vi "BMU诊断标定.vi"(5 "timeout":u32, 6 "Socket":dbl, 7 "通用配置?":bool, 8 "CAN端口":u16(ring), 9 "设备索引号":u16(ring), 10 "CAN卡类型":u32(ring)=21, 11 "从板号":u8=1) -> (3 "成功?":bool)   [LabVIEW 2013] (continued)
            n2234 = stacked-sequence {
              tunnel: w2894 -> [_ w2901 w2905]
              tunnel: w2893 -> [_ w2900 w2904]
              frame #0 {
                n2235 = local write "项目信息"(string[][] [] ("项目信息")) -> ()
              }
              frame #1 {
                n2236 = call "表格数据输入-8.6.vi"("行数"=u32 0, "列数"=u32 0, "字符串数组"=w2900, "表格引用"=w2901) -> ()  [unwired: 8 out]
              }
              frame #2 {
                n2237 = Array Size(array=w2904) -> (size(s)=w2903:i32)
                n2238 = for {
                  N: w2903 -> [_]
                  tunnel: [""] -> w2902 mode=indexing
                }
                n2239 = call "表格数据输入-8.6.vi"("行数"=u32 0, "列数"=u32 1, "字符串数组"=w2902, "表格引用"=w2905) -> ()  [unwired: 8 out]
              }
            }
          }
          event "主界面选项": Value Change {
            n2240 = event-data() -> ("NewVal"=w2909:enum32{"单选选项1", "单选选项2", "单选选项2 2", "单选选项2 3"})  [unwired: 6 out]
            n2241 = control-ref of="单选选项2 2"() -> (w2914:refnum<vi>)
            n2242 = control-ref of="单选选项2"() -> (w2916:refnum<vi>)
            n2243 = control-ref of="单选选项1"() -> (w2915:refnum<vi>)
            n2244 = control-ref of="单选选项2 3"() -> (w2910:refnum<vi>)
            n2245 = Build Array(w2915, w2916, w2914, w2910) -> (w2913:refnum<vi>[])
            n2246 = case shown="\"单选选项2 3\"" w2909 {
              selector: w2909 -> [w2927 w2932 w2937 w2942]
              tunnel: w2913 -> [w2928 w2933 w2938 w2943]
              tunnel: [w2926 w2931 w2936 w2941] -> w2919
              tunnel: [w2925 w2930 w2935 w2940] -> w2918
              tunnel: [enum32{"读写参数", "版本读取", "其它诊断"}."读写参数" ("选项卡控件 2") enum32{"读写参数", "版本读取", "其它诊断"}."版本读取" ("选项卡控件 2") enum32{"读写参数", "版本读取", "其它诊断"}."其它诊断" ("选项卡控件 2") enum32{"读写参数", "版本读取", "其它诊断", "高压板校正"}."高压板校正" ("选项卡控件 2")] -> w2917
              frame "单选选项1", Default {
                n2247 = Delete From Array(array=w2928, index=w2927) -> (deleted portion=w2925:refnum<vi>, array with subset deleted=w2926:refnum<vi>[])  [unwired: 1 in]
              }
              frame "单选选项2" {
                n2248 = Delete From Array(array=w2933, index=w2932) -> (deleted portion=w2930:refnum<vi>, array with subset deleted=w2931:refnum<vi>[])  [unwired: 1 in]
              }
              frame "单选选项2 2" {
                n2249 = Delete From Array(array=w2938, index=w2937) -> (deleted portion=w2935:refnum<vi>, array with subset deleted=w2936:refnum<vi>[])  [unwired: 1 in]
              }
              frame "单选选项2 3" {
                n2250 = Delete From Array(array=w2943, index=w2942) -> (deleted portion=w2940:refnum<vi>, array with subset deleted=w2941:refnum<vi>[])  [unwired: 1 in]
              }
            }
            n2251 = local write "面板选择"(w2917) -> ()
            n2252 = for {
              tunnel: u32 16777215 -> [w2923]
              tunnel: w2919 -> [w2922] mode=indexing
              n2253 = property class="Bool (严格)"(reference=w2922, "BoolText.TextColor"=w2923) -> ()  [unwired: 1 in, 2 out]
            }
            n2254 = property class="Bool (严格)"(reference=w2918, "BoolText.TextColor"=u32 65511) -> ()  [unwired: 1 in, 2 out]
          }
          event "主从板": Value Change {
            w2945 = FALSE ("可见")
            n2255 = event-data() -> ()  [unwired: 7 out]
            n2256 = control-ref of="单选选项2"() -> (w2953:refnum<vi>)
            n2257 = control-ref of="单选选项1"() -> (w2952:refnum<vi>)
            n2258 = local read "主从板"() -> (w2960:enum32{"单选选项2", "单选选项1"})
            n2259 = Build Array(w2953, w2952) -> (w2959:refnum<vi>[])
            n2260 = case shown="\"单选选项2\"" w2960 {
              selector: w2960 -> [w3005 w3048]
              tunnel: w2959 -> [w3006 w3047]
              tunnel: [enum32{"主板", "从板"}."主板" ("主从选择") enum32{"主板", "从板"}."从板" ("主从选择")] -> w2958
              tunnel: [w3004 w3046] -> w2955
              tunnel: [w3003 w3045] -> w2954
              tunnel: [TRUE FALSE] -> w2950
              tunnel: [w2964 w3025] -> w2947
              tunnel: [w2965 w3030] -> w2946
              tunnel: [FALSE ("可见") TRUE ("可见")] -> w2944
              frame "单选选项1", Default {
                n2261 = global read "功能码全局.vi" "主板项目信息7"() -> (w2976:bool[])
                n2262 = global read "功能码全局.vi" "主板项目信息4"() -> (w2999:bool[])
                n2263 = global read "功能码全局.vi" "主板控制类信息10"() -> (w2980:bool[])
                n2264 = global read "功能码全局.vi" "主板故障阀值9"() -> (w2977:bool[])
                n2265 = global read "功能码全局.vi" "主板项目信息5"() -> (w2990:bool[])
                n2266 = global read "功能码全局.vi" "主板项目信息6"() -> (w3000:bool[])
                n2267 = global read "功能码全局.vi" "主板版本号11"() -> (w2991:bool[])
                n2268 = Delete From Array(array=w3000, length=1 ("长度"), index=0 ("索引")) -> (deleted portion=w2989:bool[], array with subset deleted=w2972:bool[])
                n2269 = Index Array(array=w2999, index #1=5 ("索引"), index #2=6 ("索引")) -> (element #1=w2988:bool, element #2=w2971:bool)
                n2270 = Index Array(array=w2991) -> (element #1=w2984:bool, element #2=w2967:bool)  [unwired: 2 in]
                n2271 = Array Subset(array=w2977, index=2 ("索引"), length=3 ("长度")) -> (w2986:bool[])
                n2272 = Delete From Array(array=w2976, length=3 ("索引"), index=2 ("长度")) -> (deleted portion=w2987:bool[], array with subset deleted=w2970:bool[])
                n2273 = Array Subset(array=w2980, index=4 ("索引"), length=2 ("长度")) -> (w2985:bool[])
                n2274 = Delete From Array(array=w3006, index=w3005) -> (deleted portion=w3003:refnum<vi>, array with subset deleted=w3004:refnum<vi>[])  [unwired: 1 in]
                n2275 = Insert Into Array(array=w2990, new element #1=w2989, new element #2=w2988, new element #3=w2987, new element #4=w2986, new element #5=w2985, new element #6=w2984) -> (w2983:bool[])  [unwired: 1 in]
                n2276 = Array Subset(array=w2980, index=6 ("索引"), length=2 ("长度")) -> (w2968:bool[])
                n2277 = Array Subset(array=w2977, index=5 ("索引"), length=3 ("长度")) -> (w2969:bool[])
                n2278 = And Array Elements(Boolean array=w2983) -> (logical AND=w2965:bool)
                n2279 = Insert Into Array(array=w2972, new element #1=w2971, new element #2=w2970, new element #3=w2969, new element #4=w2968, new element #5=w2967) -> (w2966:bool[])  [unwired: 1 in]
                n2280 = And Array Elements(Boolean array=w2966) -> (logical AND=w2964:bool)
              }
              frame "单选选项2" {
                n2281 = global read "功能码全局.vi" "18"() -> (w3021:bool[])
                n2282 = global read "功能码全局.vi" "15"() -> (w3042:bool[])
                n2283 = global read "功能码全局.vi" "16"() -> (w3039:bool[])
                n2284 = Delete From Array(array=w3047, index=w3048) -> (deleted portion=w3045:refnum<vi>, array with subset deleted=w3046:refnum<vi>[])  [unwired: 1 in]
                n2285 = Index Array(array=w3039, index #1=4 ("索引"), index #2=5 ("索引"), index #3=6 ("索引"), index #4=7 ("索引")) -> (element #1=w3033:bool, element #2=w3032:bool, element #3=w3028:bool, element #4=w3027:bool)
                n2286 = Index Array(array=w3021, index #1=4 ("索引"), index #2=5 ("索引"), index #3=6 ("索引"), index #4=7 ("索引"), index #5=2 ("索引"), index #6=3 ("索引"), index #7=0 ("索引"), index #8=1 ("索引")) -> (element #1=w3014:bool, element #2=w3017:bool, element #3=w3016:bool, element #4=w3015:bool, element #5=w3013:bool, element #6=w3012:bool, element #7=w3007:bool, element #8=w3008:bool)
                n2287 = Delete From Array(array=w3042, length=4 ("长度"), index=0 ("索引")) -> (deleted portion=w3034:bool[], array with subset deleted=w3029:bool[])
                n2288 = Insert Into Array(array=w3029, new element #1=w3028, new element #2=w3027, new element #3=w3017, new element #4=w3016, new element #5=w3015, new element #6=w3008) -> (w3026:bool[])  [unwired: 1 in]
                n2289 = Insert Into Array(array=w3034, new element #1=w3033, new element #2=w3032, new element #3=w3014, new element #4=w3013, new element #5=w3012, new element #6=w3007) -> (w3031:bool[])  [unwired: 1 in]
                n2290 = And Array Elements(Boolean array=w3031) -> (logical AND=w3030:bool)
                n2291 = And Array Elements(Boolean array=w3026) -> (logical AND=w3025:bool)
              }
            }
            n2292 = property on="全部写入" class="Bool (严格)"("Visible"=w2947) -> ()  [unwired: 2 in, 2 out]
            n2293 = property on="全部读取" class="Bool (严格)"("Visible"=w2946) -> ()  [unwired: 2 in, 2 out]
            n2294 = property on="从板号" class="DigNum (严格)"("Visible"=w2944) -> ()  [unwired: 2 in, 2 out]
            n2295 = local write "主从选择"(w2958) -> ()
            n2296 = property on="从板个数" class="DigNum (严格)"("Visible"=w2950) -> ()  [unwired: 2 in, 2 out]
            n2297 = for {
              tunnel: u32 87470 -> [w2962]
              tunnel: w2955 -> [w2961] mode=indexing
              n2298 = property class="Bool (严格)"(reference=w2961, "BoolText.TextColor"=w2962) -> ()  [unwired: 1 in, 2 out]
            }
            n2299 = Not(x=w2950) -> (.not. x?=w2951:bool)
            n2300 = property class="Bool (严格)"(reference=w2954, "BoolText.TextColor"=u32 16777215) -> ()  [unwired: 1 in, 2 out]
            n2301 = property on="主板选项" class="Tree (严格)"("Visible"=w2950) -> ()  [unwired: 2 in, 2 out]
            n2302 = property on="从板选项" class="Tree (严格)"("Visible"=w2951) -> ()  [unwired: 2 in, 2 out]
            n2303 = property on="当前从板板号" class="DigNum (严格)"("Visible"=w2951) -> ()  [unwired: 2 in, 2 out]
            n2304 = property on="单个读取" class="Bool (严格)"("Visible"=w2945) -> ()  [unwired: 2 in, 2 out]
            n2305 = property on="单个写入" class="Bool (严格)"("Visible"=w2945) -> ()  [unwired: 2 in, 2 out]
          }
          event "从板号": Value Change {
            n2306 = event-data() -> ()  [unwired: 7 out]
            n2307 = local read "key names"() -> (w3050:string[])
            n2308 = Empty Array?(array=w3050) -> (empty?=w3049:bool)
            n2309 = case shown="假" w3049 {
              tunnel: w3050 -> [w3053 _]
              frame False {
                n2310 = stacked-sequence {
                  seq-local: [w3054 _] -> [_ w3117]
                  tunnel: w3053 -> [w3062 _]
                  frame #0 {
                    w3093 = 2 ("长度")
                    w3090 = 20 ("长度")
                    w3078 = 1 ("索引")
                    n2311 = local read "从板号"() -> (w3054:u8)
                    n2312 = local read "输出数组"() -> (w3063:string[][])
                    n2313 = Decrement(x=w3054) -> (x-1=w3060:u8)
                    n2314 = Index Array(array=w3063, index (col)=w3060) -> (element=w3091:string[])  [unwired: 1 in]
                    n2315 = global write "读配置文件全局2.vi" "从板板号"(w3054) -> ()
                    n2316 = Search 1D Array(1D array=w3062, element="风机开启温度" ("元素")) -> (index of element=w3075:i32)  [unwired: 1 in]
                    n2317 = Search 1D Array(1D array=w3062, element="电压过高一级" ("元素"), start index (0)=w3075) -> (index of element=w3073:i32)
                    n2318 = Decrement(x=w3075) -> (x-1=w3077:i32)
                    n2319 = Array Subset(array=w3091, index=w3078, length=w3077) -> (w3061:string[])
                    n2320 = Array Subset(array=w3091, index=w3073, length=21 ("长度")) -> (w3065:string[])
                    n2321 = Array Subset(array=w3062, index=w3078, length=w3077) -> (w3108:string[])
                    n2322 = Array Subset(array=w3091, index=w3075, length=7 ("长度")) -> (w3071:string[])
                    n2323 = for {
                      tunnel: w3065 -> [w3110] mode=indexing
                      tunnel: [w3109] -> w3064 mode=indexing
                      n2324 = Fract/Exp String To Number(string=w3110) -> (number=w3109:dbl)  [unwired: 3 in, 1 out]
                    }
                    n2325 = for {
                      tunnel: w3071 -> [w3112] mode=indexing
                      tunnel: [w3111] -> w3055 mode=indexing
                      n2326 = Fract/Exp String To Number(string=w3112) -> (number=w3111:dbl)  [unwired: 3 in, 1 out]
                    }
                    n2327 = Delete From Array(array=w3064, length=7 ("长度"), index=0 ("索引")) -> (deleted portion=w3058:dbl[], array with subset deleted=w3068:dbl[])
                    n2328 = Array To Cluster(array=w3055) -> (cluster=w3080:T20)
                    n2329 = global write "读配置文件全局2.vi" "加热控制参数"(w3055) -> ()
                    n2330 = Delete From Array(array=w3068, length=7 ("长度"), index=0 ("索引")) -> (deleted portion=w3057:dbl[], array with subset deleted=w3056:dbl[])
                    n2331 = local write "加热控制参数"(w3080) -> ()
                    n2332 = Array To Cluster(array=w3058) -> (cluster=w3105:T20)
                    n2333 = Array To Cluster(array=w3056) -> (cluster=w3107:T20)
                    n2334 = Array To Cluster(array=w3057) -> (cluster=w3106:T20)
                    n2335 = global write "读配置文件全局2.vi" "三级故障阀值"(w3056) -> ()
                    n2336 = global write "读配置文件全局2.vi" "一级故障阀值"(w3058) -> ()
                    n2337 = global write "读配置文件全局2.vi" "二级故障阀值"(w3057) -> ()
                    n2338 = local write "一级故障 6"(w3105) -> ()
                    n2339 = local write "一级故障 8"(w3107) -> ()
                    n2340 = local write "一级故障 7"(w3106) -> ()
                    n2341 = Search 1D Array(1D array=w3108, element="温度个数" ("元素")) -> (index of element=w3087:i32)  [unwired: 1 in]
                    n2342 = Search 1D Array(1D array=w3108, element="第一个保险通道" ("元素")) -> (index of element=w3088:i32)  [unwired: 1 in]
                    n2343 = Search 1D Array(1D array=w3108, element="电压个数" ("元素")) -> (index of element=w3086:i32)  [unwired: 1 in]
                    n2344 = Search 1D Array(1D array=w3108, element="第1通道电压个数" ("元素")) -> (index of element=w3089:i32)  [unwired: 1 in]
                    n2345 = Array Subset(array=w3061, index=w3086, length=2 ("长度")) -> (w3094:string[])
                    n2346 = Array Subset(array=w3061, index=w3087, length=w3093) -> (w3096:string[])
                    n2347 = Array Subset(array=w3061, index=w3088, length=20 ("长度")) -> (w3097:string[])
                    n2348 = Array Subset(array=w3061, index=w3089, length=w3090) -> (w3095:string[])
                    n2349 = Insert Into Array(array=w3094, new element #1=w3095, new element #2=w3096, new element #3=w3097) -> (w3059:string[])  [unwired: 1 in]
                    n2350 = Array Subset(array=w3108, index=w3086, length=w3093) -> (w3098:string[])
                    n2351 = Array Subset(array=w3108, index=w3087, length=w3093) -> (w3100:string[])
                    n2352 = Array Subset(array=w3108, index=w3088, length=w3090) -> (w3101:string[])
                    n2353 = Array Subset(array=w3108, index=w3089, length=w3090) -> (w3099:string[])
                    n2354 = global write "读配置文件全局2.vi" "表格"(w3059) -> ()
                    n2355 = Insert Into Array(array=w3098, new element #1=w3099, new element #2=w3100, new element #3=w3101) -> (w3103:string[])  [unwired: 1 in]
                    n2356 = Build Array(w3103, w3059) -> (w3102:string[][])
                    n2357 = Transpose 2D Array(2D array=w3102) -> (transposed array=w3104:string[][])
                    n2358 = local write "项目信息 2"(w3104) -> ()
                  }
                  frame #1 {
                    n2359 = Number To Decimal String(number=w3117) -> (decimal integer string=w3115:string)  [unwired: 1 in]
                    n2360 = control-ref of="结果"() -> (w3120:refnum<vi>)
                    n2361 = Concatenate Strings("从板", w3115, "导入完成") -> (w3113:string)
                    n2362 = Build Array(w3113) -> (w3118:string[])
                    n2363 = call "表格编辑.vi"("新元素/子数组"=w3118, "活动单元格:单元格背景色"=u32 6618880, "MCListbox引用句柄"=w3120) -> ()  [unwired: 9 out]
                  }
                }
              }
              frame True {
              }
            }
          }
          event "读配置文件": Value Change {
            n2364 = event-data() -> ("NewVal"=w3121:bool)  [unwired: 6 out]
            n2365 = case shown="真" w3121 {
              tunnel: w3125 -> [w3127 w3133]
              tunnel: [w3127 w3132] -> w3124
              tunnel: w3123 -> [w3126 w3131]
              tunnel: [w3126 w3130] -> w3122
              frame False {
              }
              frame True {
                n2366 = local write "布尔"(TRUE ("布尔")) -> ()
                n2367 = Enqueue Element(queue=w3133, element="读配置文件", error in (no error)=w3131) -> (queue out=w3132:refnum<queue>, error out=w3130:errorcluster)  [unwired: 2 out]
              }
            }
          }
          event "保存主板参数": Value Change {
            n2368 = event-data() -> ("NewVal"=w3134:bool)  [unwired: 6 out]
            n2369 = case shown="真" w3134 {
              tunnel: w3138 -> [w3140 w3145]
              tunnel: [w3140 w3144] -> w3137
              tunnel: w3136 -> [w3139 w3143]
              tunnel: [w3139 w3142] -> w3135
              frame False {
              }
              frame True {
                n2370 = call <vilib>:"Set Busy.vi"() -> ()  [unwired: 4 in, 8 out]
                n2371 = Enqueue Element(queue=w3145, element="写配置文件", error in (no error)=w3143) -> (queue out=w3144:refnum<queue>, error out=w3142:errorcluster)  [unwired: 2 out]
              }
            }
          }
          event "继电器全开": Value Change {
            n2372 = event-data() -> ("NewVal"=w3146:bool)  [unwired: 6 out]
            n2373 = case shown="真" w3146 {
              tunnel: w3146 -> [_ w3149]
              frame False {
              }
              frame True {
                n2374 = stacked-sequence {
                  tunnel: w3149 -> [_ w3159 _]
                  frame #0 {
                    w3150 = FALSE ("清BUFF")
                    n2375 = local write "正级继电器"(w3150) -> ()
                    n2376 = local write "负级继电器"(w3150) -> ()
                    n2377 = local write "充电继电器"(w3150) -> ()
                    n2378 = local write "加热继电器"(w3150) -> ()
                    n2379 = local write "风机继电器"(w3150) -> ()
                    n2380 = local write "预充电继电器"(w3150) -> ()
                    n2381 = local write "继电器超时处理"(FALSE ("继电器超时处理")) -> ()
                    n2382 = local write "主从选择"(enum32{"主板", "从板"}."主板" ("主从选择")) -> ()
                    n2383 = local write "清BUFF"(FALSE ("清BUFF")) -> ()
                  }
                  frame #1 {
                    n2384 = case shown="真" w3159 {
                      selector: w3159 -> [_ w3174]
                      frame False {
                      }
                      frame True {
                        w3170 = 256.0 ("y")
                        w3161 = u32 1 ("命令序号")
                        w3160 = u8 192 ("命令")
                        n2385 = local read "动作保持时间"() -> (w3171:dbl)
                        n2386 = Quotient & Remainder(x=w3171, y=w3170) -> (x-y*floor(x/y)=w3163:dbl, floor(x/y)=w3167:dbl)
                        n2387 = Quotient & Remainder(x=w3167, y=w3170) -> (x-y*floor(x/y)=w3164:dbl, floor(x/y)=w3168:dbl)
                        n2388 = Quotient & Remainder(x=w3168, y=w3170) -> (x-y*floor(x/y)=w3165:dbl, floor(x/y)=w3169:dbl)
                        n2389 = local read "设备索引号"() -> (w3178:u16)
                        n2390 = local read "CAN卡类型"() -> (w3179:u32)
                        n2391 = local read "CAN端口"() -> (w3177:u16)
                        n2392 = Boolean To (0,1)(Boolean=w3174) -> (0, 1=w3172:i16)
                        n2393 = Quotient & Remainder(x=w3169, y=w3170) -> (x-y*floor(x/y)=w3166:dbl)  [unwired: 1 out]
                        n2394 = Build Array(i16 170 ("元素"), w3172, w3166, w3165, w3164, w3163, 0.0 ("元素")) -> (w3175:dbl[])
                        n2395 = call "多帧发送机制(EV05).vi"("can卡类型"=w3179, "设备索引号"=w3178, "CAN端口"=w3177, "命令"=w3160, "板号"=u8 0, "命令序号"=w3161, "输入数据"=w3175) -> ()  [unwired: 2 in, 11 out]
                        n2396 = local write "命令序号"(w3161) -> ()
                        n2397 = local write "命令"(w3160) -> ()
                      }
                    }
                    n2398 = local write "控制1"(TRUE ("控制1")) -> ()
                    n2399 = local write "写?"(FALSE ("写?")) -> ()
                    n2400 = local write "消除"(TRUE ("消除")) -> ()
                    n2401 = global write "EV05全局变量1.vi" "流控帧 2"(TRUE ("流控帧 2")) -> ()
                    n2402 = global write "EV05全局变量1.vi" "流控帧"(FALSE ("流控帧")) -> ()
                  }
                  frame #2 {
                    n2403 = flat-sequence {
                      tunnel: [w3181] -> w3180
                      tunnel: w3180 -> [w3188]
                      frame #0 {
                        n2404 = while {
                          tunnel: [w3182] -> w3181
                          i -> [w3186]
                          stop <- w3183 stop-if-true
                          n2405 = local read "继电器超时处理"() -> (w3182:bool)
                          n2406 = Greater Or Equal?(x=w3186, y=20) -> (x >= y?=w3184:bool)
                          n2407 = Wait Until Next ms Multiple(millisecond multiple=u32 100 ("毫秒倍数")) -> ()  [unwired: 1 out]
                          n2408 = Or(x=w3182, y=w3184) -> (x .or. y?=w3183:bool)
                        }
                      }
                      frame #1 {
                        n2409 = case shown="真" w3188 {
                          frame False {
                            n2410 = One Button Dialog(message="继电器处理超时" ("消息"), button name ("OK")="是" ("按钮名称（“确定”）")) -> ()  [unwired: 1 out]
                          }
                          frame True {
                            w3191 = TRUE ("清BUFF")
                            n2411 = local write "正级继电器"(w3191) -> ()
                            n2412 = local write "负级继电器"(w3191) -> ()
                            n2413 = local write "充电继电器"(w3191) -> ()
                            n2414 = local write "加热继电器"(w3191) -> ()
                            n2415 = local write "风机继电器"(w3191) -> ()
                            n2416 = local write "预充电继电器"(w3191) -> ()
                          }
                        }
                      }
                    }
                  }
                }
              }
            }
          }
          event "继电器全关": Value Change {
            n2417 = event-data() -> ("NewVal"=w3192:bool)  [unwired: 6 out]
            n2418 = case shown="真" w3192 {
              tunnel: w3192 -> [_ w3195]
              frame False {
              }
              frame True {
                n2419 = stacked-sequence {
                  tunnel: w3195 -> [_ w3205 _]
                  frame #0 {
                    w3196 = TRUE ("清BUFF")
                    n2420 = local write "正级继电器"(w3196) -> ()
                    n2421 = local write "负级继电器"(w3196) -> ()
                    n2422 = local write "充电继电器"(w3196) -> ()
                    n2423 = local write "加热继电器"(w3196) -> ()
                    n2424 = local write "风机继电器"(w3196) -> ()
                    n2425 = local write "预充电继电器"(w3196) -> ()
                    n2426 = local write "继电器超时处理"(FALSE ("继电器超时处理")) -> ()
                    n2427 = local write "主从选择"(enum32{"主板", "从板"}."主板" ("主从选择")) -> ()
                    n2428 = global write "EV05全局变量1.vi" "流控帧"(FALSE ("流控帧")) -> ()
                    n2429 = local write "清BUFF"(FALSE ("清BUFF")) -> ()
                  }
                  frame #1 {
                    n2430 = case shown="真" w3205 {
                      selector: w3205 -> [_ w3220]
                      frame False {
                      }
                      frame True {
                        w3216 = 256.0 ("y")
                        w3207 = u32 1 ("命令序号")
                        w3206 = u8 192 ("命令")
                        n2431 = local read "动作保持时间"() -> (w3217:dbl)
                        n2432 = Quotient & Remainder(x=w3217, y=w3216) -> (x-y*floor(x/y)=w3209:dbl, floor(x/y)=w3213:dbl)
                        n2433 = Quotient & Remainder(x=w3213, y=w3216) -> (x-y*floor(x/y)=w3210:dbl, floor(x/y)=w3214:dbl)
                        n2434 = Quotient & Remainder(x=w3214, y=w3216) -> (x-y*floor(x/y)=w3211:dbl, floor(x/y)=w3215:dbl)
                        n2435 = local read "设备索引号"() -> (w3224:u16)
                        n2436 = local read "CAN卡类型"() -> (w3225:u32)
                        n2437 = local read "CAN端口"() -> (w3223:u16)
                        n2438 = Boolean To (0,1)(Boolean=w3220) -> (0, 1=w3218:i16)
                        n2439 = Quotient & Remainder(x=w3215, y=w3216) -> (x-y*floor(x/y)=w3212:dbl)  [unwired: 1 out]
                        n2440 = Build Array(i16 85 ("元素"), w3218, w3212, w3211, w3210, w3209, 0.0 ("元素")) -> (w3221:dbl[])
                        n2441 = call "多帧发送机制(EV05).vi"("can卡类型"=w3225, "设备索引号"=w3224, "CAN端口"=w3223, "命令"=w3206, "板号"=u8 0, "命令序号"=w3207, "输入数据"=w3221) -> ()  [unwired: 2 in, 11 out]
                        n2442 = local write "命令序号"(w3207) -> ()
                        n2443 = local write "命令"(w3206) -> ()
                      }
                    }
                    n2444 = local write "控制1"(TRUE ("控制1")) -> ()
                    n2445 = local write "写?"(FALSE ("写?")) -> ()
                    n2446 = local write "消除"(TRUE ("消除")) -> ()
                    n2447 = global write "EV05全局变量1.vi" "流控帧 2"(TRUE ("流控帧 2")) -> ()
                  }
                  frame #2 {
                    n2448 = flat-sequence {
                      tunnel: [w3227] -> w3226
                      tunnel: w3226 -> [w3234]
                      frame #0 {
                        n2449 = while {
                          tunnel: [w3228] -> w3227
                          i -> [w3232]
                          stop <- w3229 stop-if-true
                          n2450 = local read "继电器超时处理"() -> (w3228:bool)
                          n2451 = Greater Or Equal?(x=w3232, y=20) -> (x >= y?=w3230:bool)
                          n2452 = Wait Until Next ms Multiple(millisecond multiple=u32 100 ("毫秒倍数")) -> ()  [unwired: 1 out]
                          n2453 = Or(x=w3228, y=w3230) -> (x .or. y?=w3229:bool)
                        }
                      }
                      frame #1 {
                        n2454 = case shown="真" w3234 {
                          frame False {
                            n2455 = One Button Dialog(message="继电器处理超时" ("消息"), button name ("OK")="是" ("按钮名称（“确定”）")) -> ()  [unwired: 1 out]
                          }
                          frame True {
                            w3237 = FALSE ("清BUFF")
                            n2456 = local write "正级继电器"(w3237) -> ()
                            n2457 = local write "负级继电器"(w3237) -> ()
                            n2458 = local write "充电继电器"(w3237) -> ()
                            n2459 = local write "加热继电器"(w3237) -> ()
                            n2460 = local write "风机继电器"(w3237) -> ()
                            n2461 = local write "预充电继电器"(w3237) -> ()
                          }
                        }
                      }
                    }
                  }
                }
              }
            }
          }
          event "控制按键全为开": Value Change {
            n2462 = event-data() -> ("NewVal"=w3238:bool)  [unwired: 6 out]
            n2463 = case shown="真" w3238 {
              frame False {
              }
              frame True {
                w3239 = TRUE ("正级继电器")
                n2464 = local write "加热继电器(从)"(w3239) -> ()
                n2465 = local write "风机继电器(从)"(w3239) -> ()
                n2466 = local write "DO1 2"(w3239) -> ()
                n2467 = local write "DO1"(w3239) -> ()
                n2468 = local write "DO2"(w3239) -> ()
                n2469 = local write "正级继电器"(w3239) -> ()
                n2470 = local write "负级继电器"(w3239) -> ()
                n2471 = local write "加热继电器"(w3239) -> ()
                n2472 = local write "预充电继电器"(w3239) -> ()
                n2473 = local write "充电继电器"(w3239) -> ()
                n2474 = local write "风机继电器"(w3239) -> ()
              }
            }
          }
          event "控制按键全为关": Value Change {
            n2475 = event-data() -> ("NewVal"=w3240:bool)  [unwired: 6 out]
            n2476 = case shown="真" w3240 {
              frame False {
              }
              frame True {
                w3241 = FALSE ("正级继电器")
                n2477 = local write "加热继电器(从)"(w3241) -> ()
                n2478 = local write "风机继电器(从)"(w3241) -> ()
                n2479 = local write "DO1 2"(w3241) -> ()
                n2480 = local write "DO1"(w3241) -> ()
                n2481 = local write "DO2"(w3241) -> ()
                n2482 = local write "正级继电器"(w3241) -> ()
                n2483 = local write "负级继电器"(w3241) -> ()
                n2484 = local write "加热继电器"(w3241) -> ()
                n2485 = local write "预充电继电器"(w3241) -> ()
                n2486 = local write "充电继电器"(w3241) -> ()
                n2487 = local write "风机继电器"(w3241) -> ()
              }
            }
          }
          event "正级继电器": Value Change {
            n2488 = event-data() -> ("NewVal"=w3242:bool)  [unwired: 6 out]
            n2489 = stacked-sequence {
              tunnel: w3242 -> [_ w3255 _]
              frame #0 {
                w3245 = FALSE ("清BUFF")
                n2490 = local write "继电器超时处理"(FALSE ("继电器超时处理")) -> ()
                n2491 = local write "主从选择"(enum32{"主板", "从板"}."主板" ("主从选择")) -> ()
                n2492 = local write "正级继电器 12"(w3245) -> ()
                n2493 = local write "清BUFF"(w3245) -> ()
              }
              frame #1 {
                n2494 = case shown="假" w3255 {
                  selector: w3255 -> [w3270 w3290]
                  tunnel: [w3269 w3289] -> w3254
                  tunnel: [w3257 w3277] -> w3249
                  frame False {
                    w3265 = 256.0 ("y")
                    w3257 = u32 1 ("命令序号")
                    w3269 = u8 192 ("命令")
                    n2495 = local read "动作保持时间"() -> (w3266:dbl)
                    n2496 = Quotient & Remainder(x=w3266, y=w3265) -> (x-y*floor(x/y)=w3258:dbl, floor(x/y)=w3262:dbl)
                    n2497 = Quotient & Remainder(x=w3262, y=w3265) -> (x-y*floor(x/y)=w3259:dbl, floor(x/y)=w3263:dbl)
                    n2498 = Quotient & Remainder(x=w3263, y=w3265) -> (x-y*floor(x/y)=w3260:dbl, floor(x/y)=w3264:dbl)
                    n2499 = local read "设备索引号"() -> (w3274:u16)
                    n2500 = local read "CAN卡类型"() -> (w3275:u32)
                    n2501 = local read "CAN端口"() -> (w3273:u16)
                    n2502 = Boolean To (0,1)(Boolean=w3270) -> (0, 1=w3267:i16)
                    n2503 = Quotient & Remainder(x=w3264, y=w3265) -> (x-y*floor(x/y)=w3261:dbl)  [unwired: 1 out]
                    n2504 = Build Array(i16 1 ("元素"), w3267, w3261, w3260, w3259, w3258, 0.0 ("元素")) -> (w3271:dbl[])
                    n2505 = call "多帧发送机制(EV05).vi"("can卡类型"=w3275, "设备索引号"=w3274, "CAN端口"=w3273, "命令"=w3269, "板号"=u8 0, "命令序号"=w3257, "输入数据"=w3271) -> ()  [unwired: 2 in, 11 out]
                  }
                  frame True {
                    w3285 = 256.0 ("y")
                    w3277 = u32 1 ("命令序号")
                    w3289 = u8 192 ("命令")
                    n2506 = local read "动作保持时间"() -> (w3286:dbl)
                    n2507 = Quotient & Remainder(x=w3286, y=w3285) -> (x-y*floor(x/y)=w3278:dbl, floor(x/y)=w3282:dbl)
                    n2508 = Quotient & Remainder(x=w3282, y=w3285) -> (x-y*floor(x/y)=w3279:dbl, floor(x/y)=w3283:dbl)
                    n2509 = Quotient & Remainder(x=w3283, y=w3285) -> (x-y*floor(x/y)=w3280:dbl, floor(x/y)=w3284:dbl)
                    n2510 = local read "设备索引号"() -> (w3294:u16)
                    n2511 = local read "CAN卡类型"() -> (w3295:u32)
                    n2512 = local read "CAN端口"() -> (w3293:u16)
                    n2513 = Boolean To (0,1)(Boolean=w3290) -> (0, 1=w3287:i16)
                    n2514 = Quotient & Remainder(x=w3284, y=w3285) -> (x-y*floor(x/y)=w3281:dbl)  [unwired: 1 out]
                    n2515 = Build Array(i16 1 ("元素"), w3287, w3281, w3280, w3279, w3278, 0.0 ("元素")) -> (w3291:dbl[])
                    n2516 = call "多帧发送机制(EV05).vi"("can卡类型"=w3295, "设备索引号"=w3294, "CAN端口"=w3293, "命令"=w3289, "板号"=u8 0, "命令序号"=w3277, "输入数据"=w3291) -> ()  [unwired: 2 in, 11 out]
                  }
                }
                n2517 = local write "命令序号"(w3249) -> ()
                n2518 = local write "命令"(w3254) -> ()
                n2519 = local write "控制1"(TRUE ("控制1")) -> ()
                n2520 = local write "写?"(FALSE ("写?")) -> ()
                n2521 = global write "EV05全局变量1.vi" "流控帧"(FALSE ("流控帧")) -> ()
                n2522 = local write "消除"(TRUE ("消除")) -> ()
                n2523 = global write "EV05全局变量1.vi" "流控帧 2"(TRUE ("流控帧 2")) -> ()
              }
              frame #2 {
                n2524 = flat-sequence {
                  tunnel: [w3297] -> w3296
                  tunnel: w3296 -> [w3304]
                  frame #0 {
                    n2525 = while {
                      tunnel: [w3298] -> w3297
                      i -> [w3302]
                      stop <- w3299 stop-if-true
                      n2526 = local read "继电器超时处理"() -> (w3298:bool)
                      n2527 = Greater Or Equal?(x=w3302, y=20) -> (x >= y?=w3300:bool)
                      n2528 = Wait Until Next ms Multiple(millisecond multiple=u32 100 ("毫秒倍数")) -> ()  [unwired: 1 out]
                      n2529 = Or(x=w3298, y=w3300) -> (x .or. y?=w3299:bool)
                    }
                  }
                  frame #1 {
                    n2530 = case shown="假" w3304 {
                      frame False {
                        n2531 = local read "正级继电器"() -> (w3306:bool)
                        n2532 = Not(x=w3306) -> (.not. x?=w3305:bool)
                        n2533 = local write "正级继电器"(w3305) -> ()
                        n2534 = One Button Dialog(message="继电器处理超时" ("消息"), button name ("OK")="是" ("按钮名称（“确定”）")) -> ()  [unwired: 1 out]
                      }
                      frame True {
                      }
                    }
                  }
                }
              }
            }
          }
          event "负级继电器": Value Change {
            n2535 = event-data() -> ("NewVal"=w3309:bool)  [unwired: 6 out]
            n2536 = stacked-sequence {
              tunnel: w3309 -> [_ w3322 _]
              frame #0 {
                w3312 = FALSE ("继电器超时处理")
                n2537 = local write "继电器超时处理"(w3312) -> ()
                n2538 = local write "正级继电器 2"(w3312) -> ()
                n2539 = local write "主从选择"(enum32{"主板", "从板"}."主板" ("主从选择")) -> ()
              }
              frame #1 {
                n2540 = case shown="假" w3322 {
                  selector: w3322 -> [w3336 w3356]
                  tunnel: [w3335 w3355] -> w3321
                  tunnel: [w3324 w3344] -> w3316
                  frame False {
                    w3332 = 256.0 ("y")
                    w3324 = u32 1 ("命令序号")
                    w3335 = u8 192 ("命令")
                    n2541 = local read "动作保持时间"() -> (w3333:dbl)
                    n2542 = Quotient & Remainder(x=w3333, y=w3332) -> (x-y*floor(x/y)=w3325:dbl, floor(x/y)=w3329:dbl)
                    n2543 = Quotient & Remainder(x=w3329, y=w3332) -> (x-y*floor(x/y)=w3326:dbl, floor(x/y)=w3330:dbl)
                    n2544 = Quotient & Remainder(x=w3330, y=w3332) -> (x-y*floor(x/y)=w3327:dbl, floor(x/y)=w3331:dbl)
                    n2545 = Quotient & Remainder(x=w3331, y=w3332) -> (x-y*floor(x/y)=w3328:dbl)  [unwired: 1 out]
                    n2546 = Boolean To (0,1)(Boolean=w3336) -> (0, 1=w3334:i16)
                    n2547 = local read "设备索引号"() -> (w3341:u16)
                    n2548 = local read "CAN卡类型"() -> (w3342:u32)
                    n2549 = local read "CAN端口"() -> (w3340:u16)
                    n2550 = Build Array(i16 2 ("元素"), w3334, w3328, w3327, w3326, w3325, 0.0 ("元素")) -> (w3338:dbl[])
                    n2551 = call "多帧发送机制(EV05).vi"("can卡类型"=w3342, "设备索引号"=w3341, "CAN端口"=w3340, "命令"=w3335, "板号"=u8 0, "命令序号"=w3324, "输入数据"=w3338) -> ()  [unwired: 2 in, 11 out]
                  }
                  frame True {
                    w3352 = 256.0 ("y")
                    w3344 = u32 1 ("命令序号")
                    w3355 = u8 192 ("命令")
                    n2552 = local read "动作保持时间"() -> (w3353:dbl)
                    n2553 = Quotient & Remainder(x=w3353, y=w3352) -> (x-y*floor(x/y)=w3345:dbl, floor(x/y)=w3349:dbl)
                    n2554 = Quotient & Remainder(x=w3349, y=w3352) -> (x-y*floor(x/y)=w3346:dbl, floor(x/y)=w3350:dbl)
                    n2555 = Quotient & Remainder(x=w3350, y=w3352) -> (x-y*floor(x/y)=w3347:dbl, floor(x/y)=w3351:dbl)
                    n2556 = Quotient & Remainder(x=w3351, y=w3352) -> (x-y*floor(x/y)=w3348:dbl)  [unwired: 1 out]
                    n2557 = Boolean To (0,1)(Boolean=w3356) -> (0, 1=w3354:i16)
                    n2558 = local read "设备索引号"() -> (w3361:u16)
                    n2559 = local read "CAN卡类型"() -> (w3362:u32)
                    n2560 = local read "CAN端口"() -> (w3360:u16)
                    n2561 = Build Array(i16 2 ("元素"), w3354, w3348, w3347, w3346, w3345, 0.0 ("元素")) -> (w3358:dbl[])
                    n2562 = call "多帧发送机制(EV05).vi"("can卡类型"=w3362, "设备索引号"=w3361, "CAN端口"=w3360, "命令"=w3355, "板号"=u8 0, "命令序号"=w3344, "输入数据"=w3358) -> ()  [unwired: 2 in, 11 out]
                  }
                }
                n2563 = local write "命令"(w3321) -> ()
                n2564 = local write "命令序号"(w3316) -> ()
                n2565 = local write "清BUFF"(FALSE ("清BUFF")) -> ()
                n2566 = global write "EV05全局变量1.vi" "流控帧"(FALSE ("流控帧")) -> ()
                n2567 = local write "控制1"(TRUE ("控制1")) -> ()
                n2568 = global write "EV05全局变量1.vi" "流控帧 2"(TRUE ("流控帧 2")) -> ()
                n2569 = local write "写?"(FALSE ("写?")) -> ()
                n2570 = local write "消除"(TRUE ("消除")) -> ()
              }
              frame #2 {
                n2571 = flat-sequence {
                  tunnel: [w3364] -> w3363
                  tunnel: w3363 -> [w3371]
                  frame #0 {
                    n2572 = while {
                      tunnel: [w3365] -> w3364
                      i -> [w3369]
                      stop <- w3366 stop-if-true
                      n2573 = local read "继电器超时处理"() -> (w3365:bool)
                      n2574 = Greater Or Equal?(x=w3369, y=20) -> (x >= y?=w3367:bool)
                      n2575 = Wait Until Next ms Multiple(millisecond multiple=u32 100 ("毫秒倍数")) -> ()  [unwired: 1 out]
                      n2576 = Or(x=w3365, y=w3367) -> (x .or. y?=w3366:bool)
                    }
                  }
                  frame #1 {
                    n2577 = case shown="假" w3371 {
                      frame False {
                        n2578 = local read "负级继电器"() -> (w3372:bool)
                        n2579 = Not(x=w3372) -> (.not. x?=w3373:bool)
                        n2580 = local write "负级继电器"(w3373) -> ()
                        n2581 = One Button Dialog(message="继电器处理超时" ("消息"), button name ("OK")="是" ("按钮名称（“确定”）")) -> ()  [unwired: 1 out]
                      }
                      frame True {
                      }
                    }
                  }
                }
              }
            }
          }
          event "预充电继电器": Value Change {
            n2582 = event-data() -> ("NewVal"=w3376:bool)  [unwired: 6 out]
            n2583 = stacked-sequence {
              tunnel: w3376 -> [_ w3389 _]
              frame #0 {
                w3380 = FALSE ("继电器超时处理")
                n2584 = local write "继电器超时处理"(w3380) -> ()
                n2585 = local write "正级继电器 3"(w3380) -> ()
                n2586 = global write "EV05全局变量1.vi" "流控帧"(FALSE ("流控帧")) -> ()
                n2587 = local write "主从选择"(enum32{"主板", "从板"}."主板" ("主从选择")) -> ()
              }
              frame #1 {
                n2588 = case shown="假" w3389 {
                  selector: w3389 -> [w3403 w3423]
                  tunnel: [w3402 w3422] -> w3388
                  tunnel: [w3391 w3411] -> w3383
                  frame False {
                    w3399 = 256.0 ("y")
                    w3391 = u32 1 ("命令序号")
                    w3402 = u8 192 ("命令")
                    n2589 = local read "动作保持时间"() -> (w3400:dbl)
                    n2590 = Quotient & Remainder(x=w3400, y=w3399) -> (x-y*floor(x/y)=w3392:dbl, floor(x/y)=w3396:dbl)
                    n2591 = Quotient & Remainder(x=w3396, y=w3399) -> (x-y*floor(x/y)=w3393:dbl, floor(x/y)=w3397:dbl)
                    n2592 = Quotient & Remainder(x=w3397, y=w3399) -> (x-y*floor(x/y)=w3394:dbl, floor(x/y)=w3398:dbl)
                    n2593 = Quotient & Remainder(x=w3398, y=w3399) -> (x-y*floor(x/y)=w3395:dbl)  [unwired: 1 out]
                    n2594 = Boolean To (0,1)(Boolean=w3403) -> (0, 1=w3401:i16)
                    n2595 = local read "设备索引号"() -> (w3408:u16)
                    n2596 = local read "CAN卡类型"() -> (w3409:u32)
                    n2597 = local read "CAN端口"() -> (w3407:u16)
                    n2598 = Build Array(i16 3 ("元素"), w3401, w3395, w3394, w3393, w3392, 0.0 ("元素")) -> (w3405:dbl[])
                    n2599 = call "多帧发送机制(EV05).vi"("can卡类型"=w3409, "设备索引号"=w3408, "CAN端口"=w3407, "命令"=w3402, "板号"=u8 0, "命令序号"=w3391, "输入数据"=w3405) -> ()  [unwired: 2 in, 11 out]
                  }
                  frame True {
                    w3419 = 256.0 ("y")
                    w3411 = u32 1 ("命令序号")
                    w3422 = u8 192 ("命令")
                    n2600 = local read "动作保持时间"() -> (w3420:dbl)
                    n2601 = Quotient & Remainder(x=w3420, y=w3419) -> (x-y*floor(x/y)=w3412:dbl, floor(x/y)=w3416:dbl)
                    n2602 = Quotient & Remainder(x=w3416, y=w3419) -> (x-y*floor(x/y)=w3413:dbl, floor(x/y)=w3417:dbl)
                    n2603 = Quotient & Remainder(x=w3417, y=w3419) -> (x-y*floor(x/y)=w3414:dbl, floor(x/y)=w3418:dbl)
                    n2604 = Quotient & Remainder(x=w3418, y=w3419) -> (x-y*floor(x/y)=w3415:dbl)  [unwired: 1 out]
                    n2605 = Boolean To (0,1)(Boolean=w3423) -> (0, 1=w3421:i16)
                    n2606 = local read "设备索引号"() -> (w3428:u16)
                    n2607 = local read "CAN卡类型"() -> (w3429:u32)
                    n2608 = local read "CAN端口"() -> (w3427:u16)
                    n2609 = Build Array(i16 3 ("元素"), w3421, w3415, w3414, w3413, w3412, 0.0 ("元素")) -> (w3425:dbl[])
                    n2610 = call "多帧发送机制(EV05).vi"("can卡类型"=w3429, "设备索引号"=w3428, "CAN端口"=w3427, "命令"=w3422, "板号"=u8 0, "命令序号"=w3411, "输入数据"=w3425) -> ()  [unwired: 2 in, 11 out]
                  }
                }
                n2611 = local write "命令序号"(w3383) -> ()
                n2612 = local write "清BUFF"(FALSE ("清BUFF")) -> ()
                n2613 = local write "控制1"(TRUE ("控制1")) -> ()
                n2614 = global write "EV05全局变量1.vi" "流控帧 2"(TRUE ("流控帧 2")) -> ()
                n2615 = local write "消除"(TRUE ("消除")) -> ()
                n2616 = local write "命令"(w3388) -> ()
                n2617 = local write "写?"(FALSE ("写?")) -> ()
              }
              frame #2 {
                n2618 = flat-sequence {
                  tunnel: [w3431] -> w3430
                  tunnel: w3430 -> [w3438]
                  frame #0 {
                    n2619 = while {
                      tunnel: [w3432] -> w3431
                      i -> [w3436]
                      stop <- w3433 stop-if-true
                      n2620 = local read "继电器超时处理"() -> (w3432:bool)
                      n2621 = Greater Or Equal?(x=w3436, y=20) -> (x >= y?=w3434:bool)
                      n2622 = Wait Until Next ms Multiple(millisecond multiple=u32 100 ("毫秒倍数")) -> ()  [unwired: 1 out]
                      n2623 = Or(x=w3432, y=w3434) -> (x .or. y?=w3433:bool)
                    }
                  }
                  frame #1 {
                    n2624 = case shown="假" w3438 {
                      frame False {
                        n2625 = local read "预充电继电器"() -> (w3439:bool)
                        n2626 = Not(x=w3439) -> (.not. x?=w3440:bool)
                        n2627 = local write "预充电继电器"(w3440) -> ()
                        n2628 = One Button Dialog(message="继电器处理超时" ("消息"), button name ("OK")="是" ("按钮名称（“确定”）")) -> ()  [unwired: 1 out]
                      }
                      frame True {
                      }
                    }
                  }
                }
              }
            }
          }
          event "加热继电器": Value Change {
            n2629 = event-data() -> ("NewVal"=w3443:bool)  [unwired: 6 out]
            n2630 = stacked-sequence {
              tunnel: w3443 -> [_ w3456 _]
              frame #0 {
                w3447 = FALSE ("继电器超时处理")
                n2631 = local write "继电器超时处理"(w3447) -> ()
                n2632 = local write "正级继电器 5"(w3447) -> ()
                n2633 = global write "EV05全局变量1.vi" "流控帧"(FALSE ("流控帧")) -> ()
                n2634 = local write "主从选择"(enum32{"主板", "从板"}."主板" ("主从选择")) -> ()
              }
              frame #1 {
                n2635 = case shown="假" w3456 {
                  selector: w3456 -> [w3470 w3490]
                  tunnel: [w3469 w3489] -> w3455
                  tunnel: [w3458 w3478] -> w3450
                  frame False {
                    w3466 = 256.0 ("y")
                    w3458 = u32 1 ("命令序号")
                    w3469 = u8 192 ("命令")
                    n2636 = local read "动作保持时间"() -> (w3467:dbl)
                    n2637 = Quotient & Remainder(x=w3467, y=w3466) -> (x-y*floor(x/y)=w3459:dbl, floor(x/y)=w3463:dbl)
                    n2638 = Quotient & Remainder(x=w3463, y=w3466) -> (x-y*floor(x/y)=w3460:dbl, floor(x/y)=w3464:dbl)
                    n2639 = Quotient & Remainder(x=w3464, y=w3466) -> (x-y*floor(x/y)=w3461:dbl, floor(x/y)=w3465:dbl)
                    n2640 = Quotient & Remainder(x=w3465, y=w3466) -> (x-y*floor(x/y)=w3462:dbl)  [unwired: 1 out]
                    n2641 = Boolean To (0,1)(Boolean=w3470) -> (0, 1=w3468:i16)
                    n2642 = local read "设备索引号"() -> (w3475:u16)
                    n2643 = local read "CAN卡类型"() -> (w3476:u32)
                    n2644 = local read "CAN端口"() -> (w3474:u16)
                    n2645 = Build Array(i16 4 ("元素"), w3468, w3462, w3461, w3460, w3459, 0.0 ("元素")) -> (w3472:dbl[])
                    n2646 = call "多帧发送机制(EV05).vi"("can卡类型"=w3476, "设备索引号"=w3475, "CAN端口"=w3474, "命令"=w3469, "板号"=u8 0, "命令序号"=w3458, "输入数据"=w3472) -> ()  [unwired: 2 in, 11 out]
                  }
                  frame True {
                    w3486 = 256.0 ("y")
                    w3478 = u32 1 ("命令序号")
                    w3489 = u8 192 ("命令")
                    n2647 = local read "动作保持时间"() -> (w3487:dbl)
                    n2648 = Quotient & Remainder(x=w3487, y=w3486) -> (x-y*floor(x/y)=w3479:dbl, floor(x/y)=w3483:dbl)
                    n2649 = Quotient & Remainder(x=w3483, y=w3486) -> (x-y*floor(x/y)=w3480:dbl, floor(x/y)=w3484:dbl)
                    n2650 = Quotient & Remainder(x=w3484, y=w3486) -> (x-y*floor(x/y)=w3481:dbl, floor(x/y)=w3485:dbl)
                    n2651 = Quotient & Remainder(x=w3485, y=w3486) -> (x-y*floor(x/y)=w3482:dbl)  [unwired: 1 out]
                    n2652 = Boolean To (0,1)(Boolean=w3490) -> (0, 1=w3488:i16)
                    n2653 = local read "设备索引号"() -> (w3495:u16)
                    n2654 = local read "CAN卡类型"() -> (w3496:u32)
                    n2655 = local read "CAN端口"() -> (w3494:u16)
                    n2656 = Build Array(i16 4 ("元素"), w3488, w3482, w3481, w3480, w3479, 0.0 ("元素")) -> (w3492:dbl[])
                    n2657 = call "多帧发送机制(EV05).vi"("can卡类型"=w3496, "设备索引号"=w3495, "CAN端口"=w3494, "命令"=w3489, "板号"=u8 0, "命令序号"=w3478, "输入数据"=w3492) -> ()  [unwired: 2 in, 11 out]
                  }
                }
                n2658 = local write "命令序号"(w3450) -> ()
                n2659 = local write "清BUFF"(FALSE ("清BUFF")) -> ()
                n2660 = local write "命令"(w3455) -> ()
                n2661 = local write "控制1"(TRUE ("控制1")) -> ()
                n2662 = local write "写?"(FALSE ("写?")) -> ()
                n2663 = global write "EV05全局变量1.vi" "流控帧 2"(TRUE ("流控帧 2")) -> ()
                n2664 = local write "消除"(TRUE ("消除")) -> ()
              }
              frame #2 {
                n2665 = flat-sequence {
                  tunnel: [w3498] -> w3497
                  tunnel: w3497 -> [w3505]
                  frame #0 {
                    n2666 = while {
                      tunnel: [w3499] -> w3498
                      i -> [w3503]
                      stop <- w3500 stop-if-true
                      n2667 = local read "继电器超时处理"() -> (w3499:bool)
                      n2668 = Greater Or Equal?(x=w3503, y=20) -> (x >= y?=w3501:bool)
                      n2669 = Wait Until Next ms Multiple(millisecond multiple=u32 100 ("毫秒倍数")) -> ()  [unwired: 1 out]
                      n2670 = Or(x=w3499, y=w3501) -> (x .or. y?=w3500:bool)
                    }
                  }
                  frame #1 {
                    n2671 = case shown="假" w3505 {
                      frame False {
                        n2672 = local read "加热继电器"() -> (w3506:bool)
                        n2673 = Not(x=w3506) -> (.not. x?=w3507:bool)
                        n2674 = local write "加热继电器"(w3507) -> ()
                        n2675 = One Button Dialog(message="继电器处理超时" ("消息"), button name ("OK")="是" ("按钮名称（“确定”）")) -> ()  [unwired: 1 out]
                      }
                      frame True {
                      }
                    }
                  }
                }
              }
            }
          }
          event "充电继电器": Value Change {
            n2676 = event-data() -> ("NewVal"=w3510:bool)  [unwired: 6 out]
            n2677 = stacked-sequence {
              tunnel: w3510 -> [_ w3523 _]
              frame #0 {
                w3514 = FALSE ("继电器超时处理")
                n2678 = local write "主从选择"(enum32{"主板", "从板"}."主板" ("主从选择")) -> ()
                n2679 = global write "EV05全局变量1.vi" "流控帧"(FALSE ("流控帧")) -> ()
                n2680 = local write "继电器超时处理"(w3514) -> ()
                n2681 = local write "正级继电器 4"(w3514) -> ()
              }
              frame #1 {
                n2682 = case shown="假" w3523 {
                  selector: w3523 -> [w3537 w3557]
                  tunnel: [w3536 w3556] -> w3522
                  tunnel: [w3525 w3545] -> w3517
                  frame False {
                    w3533 = 256.0 ("y")
                    w3525 = u32 1 ("命令序号")
                    w3536 = u8 192 ("命令")
                    n2683 = local read "动作保持时间"() -> (w3534:dbl)
                    n2684 = Quotient & Remainder(x=w3534, y=w3533) -> (x-y*floor(x/y)=w3526:dbl, floor(x/y)=w3530:dbl)
                    n2685 = Quotient & Remainder(x=w3530, y=w3533) -> (x-y*floor(x/y)=w3527:dbl, floor(x/y)=w3531:dbl)
                    n2686 = Quotient & Remainder(x=w3531, y=w3533) -> (x-y*floor(x/y)=w3528:dbl, floor(x/y)=w3532:dbl)
                    n2687 = Quotient & Remainder(x=w3532, y=w3533) -> (x-y*floor(x/y)=w3529:dbl)  [unwired: 1 out]
                    n2688 = Boolean To (0,1)(Boolean=w3537) -> (0, 1=w3535:i16)
                    n2689 = local read "设备索引号"() -> (w3542:u16)
                    n2690 = local read "CAN卡类型"() -> (w3543:u32)
                    n2691 = local read "CAN端口"() -> (w3541:u16)
                    n2692 = Build Array(i16 5 ("元素"), w3535, w3529, w3528, w3527, w3526, 0.0 ("元素")) -> (w3539:dbl[])
                    n2693 = call "多帧发送机制(EV05).vi"("can卡类型"=w3543, "设备索引号"=w3542, "CAN端口"=w3541, "命令"=w3536, "板号"=u8 0, "命令序号"=w3525, "输入数据"=w3539) -> ()  [unwired: 2 in, 11 out]
                  }
                  frame True {
                    w3553 = 256.0 ("y")
                    w3545 = u32 1 ("命令序号")
                    w3556 = u8 192 ("命令")
                    n2694 = local read "动作保持时间"() -> (w3554:dbl)
                    n2695 = Quotient & Remainder(x=w3554, y=w3553) -> (x-y*floor(x/y)=w3546:dbl, floor(x/y)=w3550:dbl)
                    n2696 = Quotient & Remainder(x=w3550, y=w3553) -> (x-y*floor(x/y)=w3547:dbl, floor(x/y)=w3551:dbl)
                    n2697 = Quotient & Remainder(x=w3551, y=w3553) -> (x-y*floor(x/y)=w3548:dbl, floor(x/y)=w3552:dbl)
                    n2698 = Quotient & Remainder(x=w3552, y=w3553) -> (x-y*floor(x/y)=w3549:dbl)  [unwired: 1 out]
                    n2699 = Boolean To (0,1)(Boolean=w3557) -> (0, 1=w3555:i16)
                    n2700 = local read "设备索引号"() -> (w3562:u16)
                    n2701 = local read "CAN卡类型"() -> (w3563:u32)
                    n2702 = local read "CAN端口"() -> (w3561:u16)
                    n2703 = Build Array(i16 5 ("元素"), w3555, w3549, w3548, w3547, w3546, 0.0 ("元素")) -> (w3559:dbl[])
                    n2704 = call "多帧发送机制(EV05).vi"("can卡类型"=w3563, "设备索引号"=w3562, "CAN端口"=w3561, "命令"=w3556, "板号"=u8 0, "命令序号"=w3545, "输入数据"=w3559) -> ()  [unwired: 2 in, 11 out]
                  }
                }
                n2705 = local write "命令序号"(w3517) -> ()
                n2706 = local write "命令"(w3522) -> ()
                n2707 = local write "清BUFF"(FALSE ("清BUFF")) -> ()
                n2708 = local write "控制1"(TRUE ("控制1")) -> ()
                n2709 = global write "EV05全局变量1.vi" "流控帧 2"(TRUE ("流控帧 2")) -> ()
                n2710 = local write "写?"(FALSE ("写?")) -> ()
                n2711 = local write "消除"(TRUE ("消除")) -> ()
              }
              frame #2 {
                n2712 = flat-sequence {
                  tunnel: [w3565] -> w3564
                  tunnel: w3564 -> [w3572]
                  frame #0 {
                    n2713 = while {
                      tunnel: [w3566] -> w3565
                      i -> [w3570]
                      stop <- w3567 stop-if-true
                      n2714 = local read "继电器超时处理"() -> (w3566:bool)
                      n2715 = Greater Or Equal?(x=w3570, y=20) -> (x >= y?=w3568:bool)
                      n2716 = Wait Until Next ms Multiple(millisecond multiple=u32 100 ("毫秒倍数")) -> ()  [unwired: 1 out]
                      n2717 = Or(x=w3566, y=w3568) -> (x .or. y?=w3567:bool)
                    }
                  }
                  frame #1 {
                    n2718 = case shown="假" w3572 {
                      frame False {
                        n2719 = local read "充电继电器"() -> (w3573:bool)
                        n2720 = Not(x=w3573) -> (.not. x?=w3574:bool)
                        n2721 = local write "充电继电器"(w3574) -> ()
                        n2722 = One Button Dialog(message="继电器处理超时" ("消息"), button name ("OK")="是" ("按钮名称（“确定”）")) -> ()  [unwired: 1 out]
                      }
